vi "SMGR_intercom_01.vi"(8 "error in (no error)":errorcluster, 11 "URL:port":string="ssh.alwaysdata.com:12673") -> (0 "error out":errorcluster)   [LabVIEW 2010]
panel:
  in  "InputData":T1
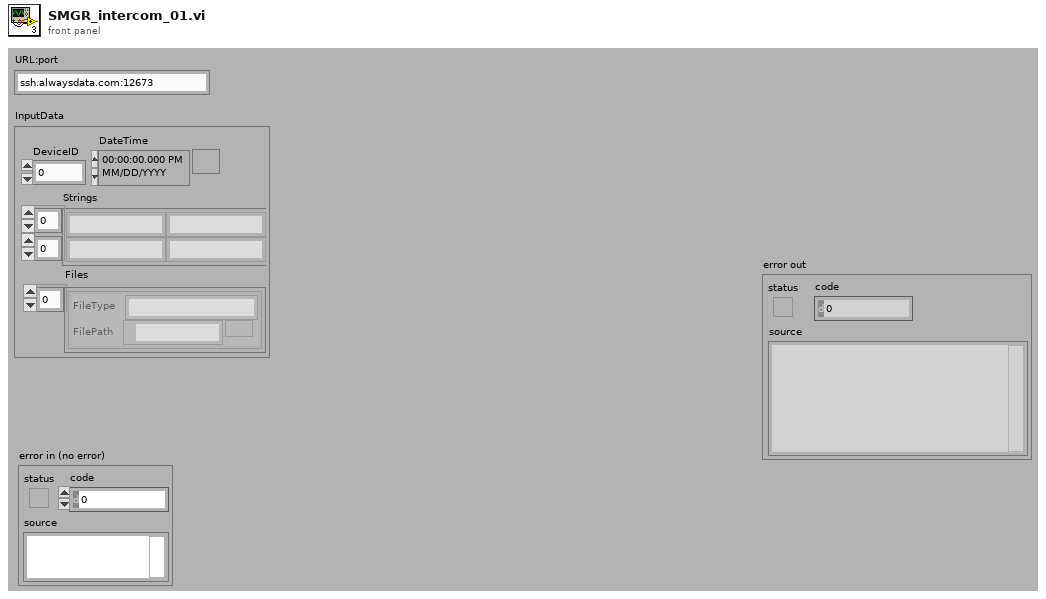
[diagram p1: front panel]
types:
  T1 = cluster{"DeviceID":i32, "DateTime":timestamp, "Files":cluster{"FileType":string, "FilePath":path}[], "Strings":string[][]}
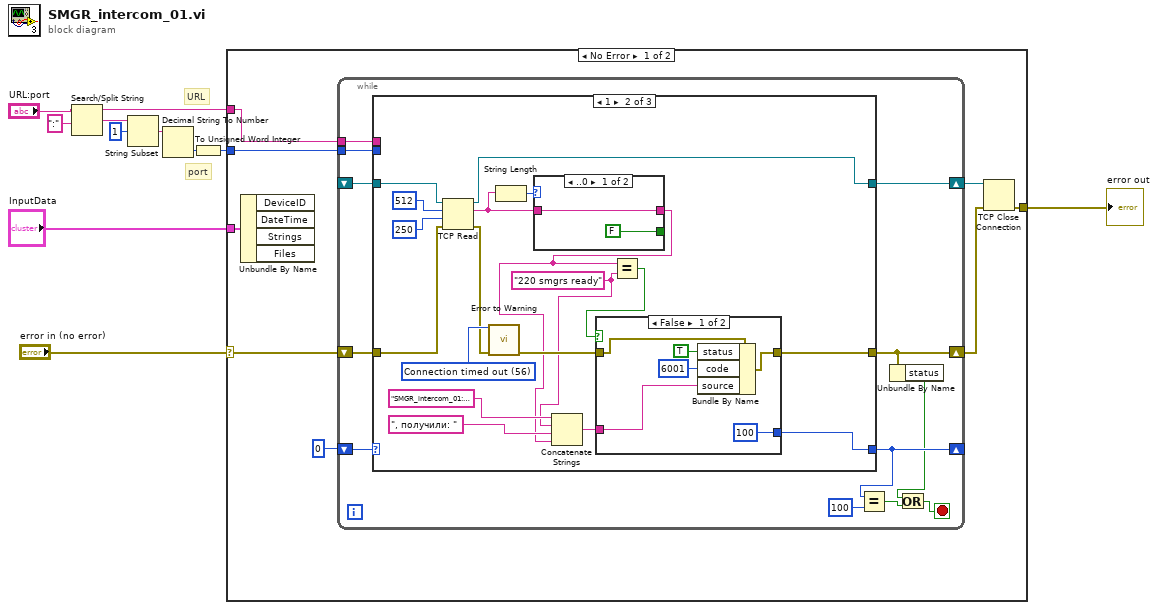
[diagram p0: block diagram]
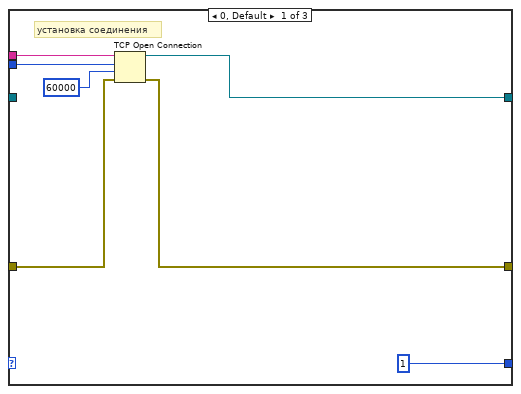
[diagram p2: hidden frame]
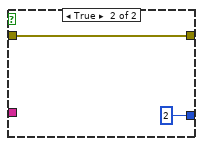
[diagram p3: hidden frame]
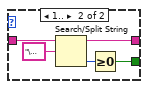
[diagram p4: hidden frame]
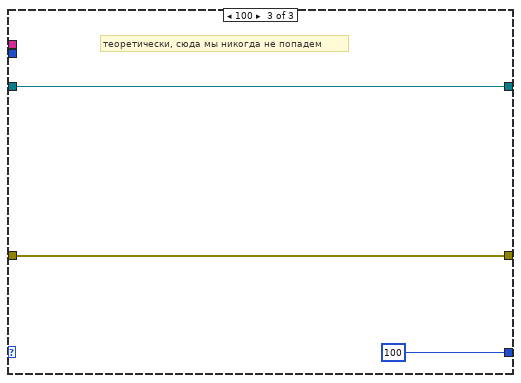
[diagram p5: hidden frame]
diagram:
  # "port"
  # "URL"
  n1 = Search/Split String(string="URL:port", search string/char (-)=":") -> (substring before match=w5:string, match + rest of string=w8:string)  [unwired: 1 in, 1 out]
  n2 = String Subset(string=w8, offset (0)=1) -> (substring=w9:string)  [unwired: 1 in]
  n3 = Decimal String To Number(string=w9) -> (number=w4:i32)  [unwired: 2 in, 1 out]
  n4 = To Unsigned Word Integer(number=w4) -> (unsigned 16bit integer=w2:u16)
  n5 = case shown="No Error" "error in (no error)" {
    selector: "error in (no error)" -> [w18 w75]
    tunnel: w5 -> [w16 _]
    tunnel: w2 -> [w15 _]
    tunnel: "InputData" -> [w19 _]
    tunnel: [w12 w75] -> w1
    frame No Error {
      n6 = Unbundle By Name(w19) -> ()  [unwired: 4 out]
      n7 = while {
        shift-right: [w24] -> _
        shift-left: 0 -> [w31]
        tunnel: w16 -> [w30]
        tunnel: w15 -> [w29]
        shift-right: [w21] -> w13
        shift-left: w18 -> [w28]
        shift-right: [w27] -> w14
        shift-left: _ -> [w26]
        stop <- w23 stop-if-true
        n8 = case shown="1" w31 {
          tunnel: [1 w44 100] -> w24
          tunnel: w30 -> [w37 _ _]
          tunnel: w29 -> [w36 _ _]
          tunnel: w28 -> [w35 w54 w74]
          tunnel: [w34 w45 w74] -> w21
          tunnel: [w32 w55 w72] -> w27
          tunnel: w26 -> [_ w56 w72]
          frame 0, Default {
            # "установка соединения"
            n9 = TCP Open Connection(address=w37, remote port or service name=w36, timeout ms (60000)=60000, error in (no error)=w35) -> (connection ID=w32:refnum<k5>, error out=w34:errorcluster)  [unwired: 1 in]
          }
          frame 1 {
            w42 = "220 smgrs ready"
            w51 = 56 items=["No Error", "Argument Error", "Memory Full", "Out of Zone", "End of File", "File Already Open", "Generic File IO Error", "File Not Found", "File Permission Error", "Disk Full", "Duplicate Path", "Too Many Files Open", "Not Enabled", "Resource File Not Found", "Cannot Add Resource", "Resource Not Found", "Image Not Found", "Image Memory Error", "Pen Does Not Exist", "Config Bad Type", "Config Token Not Found", "Config Parse Error", "Config Memory Error", "Bad External Code Format", "Bad External Code Offset", "External Code Not Present", "Null Window", "Destroy Window Mixup", "Null Menu", "Print Aborted", "Bad Print Record", "Print Driver Error", "Windows Error During Print", "Memory Error During Print", "Print Dialog Error", "Generic Print Error", "Invalid Device Refnum", "Device Not Found", "Device Parameter Error", "Device Unit Error", "Can't Open Device", "Device Call Aborted", "Generic Error", "Cancelled By User", "Object ID Too Low", "Object ID Too High", "Object Not In Heap", "Unknown Heap", "Bad DefProc ID", "DefProc Not In Table", "Message Out Of Range", "Null Method", "Unknown Message", "Manager Call Not Supported", "Bad address", "Connection In progress", "Connection timed out", "Connection is already in progress", "Network attribute not supported", "Network error", "Address in use", "System out of memory", "Connection aborted", "Connection refused", "Connection is not connected", "Connection is already connected", "Connection closed", "Initialize error (interapplication manager)", "Bad occurrence", "Wait on unbound occurrence handler", "Occurrence queue overflow", "Bad path", "Semaphore not signaled", "Unrecognized type (interapplication manager)"] ("1st Error to Convert")
            n10 = TCP Read(connection ID=w56, bytes to read=512, error in (no error)=w54, 9:250 ("timeout ms (25000)")) -> (connection ID out=w55:refnum<k5>, data out=w48:string, error out=w50:errorcluster)  [unwired: 1 in]
            n11 = call <vilib>:"Error to Warning.vi"("1st Error to Convert"=w51, "error in"=w50) -> ("warning out"=w47:errorcluster)  [unwired: 13 in]
            n12 = String Length(string=w48) -> (length=w49:i32)
            n13 = case shown="..0" w49 {
              tunnel: w48 -> [w65 w70]
              tunnel: [w65 w67] -> w40
              tunnel: [FALSE w68] -> _
              frame ..0 {
              }
              frame 1.. {
                n14 = Search/Split String(string=w70, search string/char (-)="\u0004") -> (substring before match=w67:string, offset of match=w69:i32)  [unwired: 1 in, 1 out]
                n15 = Greater Or Equal To 0?(x=w69) -> (x >= 0?=w68:bool)
              }
            }
            n16 = Concatenate Strings("SMGR_intercom_01: ожидали получить ", w42, ", получили: ", w40) -> (w39:string)
            n17 = Equal?(x=w40, y=w42) -> (x = y?=w46:bool)
            n18 = case shown="False" w46 {
              tunnel: w47 -> [w60 w64]
              tunnel: [w61 w64] -> w45
              tunnel: [100 2] -> w44
              tunnel: w39 -> [w57 _]
              frame False {
                n19 = Bundle By Name(cluster=w60, "status"=TRUE, "code"=6001, "source"=w57) -> (w61:errorcluster)
              }
              frame True {
              }
            }
          }
          frame 100 {
            # "теоретически, сюда мы никогда не попадем"
          }
        }
        n20 = Equal?(x=w24, y=100) -> (x = y?=w22:bool)
        n21 = Unbundle By Name(w21) -> ("status"=w20:bool)
        n22 = Or(x=w20, y=w22) -> (x .or. y?=w23:bool)
      }
      n23 = TCP Close Connection(connection ID=w14, error in (no error)=w13) -> (error out=w12:errorcluster)  [unwired: 1 in, 1 out]
    }
    frame Error {
    }
  }
  "error out" <- w1
